vi "Pot to Degrees.vi"(11 "Pot Value":dbl) -> (3 "Degrees":dbl)   [LabVIEW 2015]
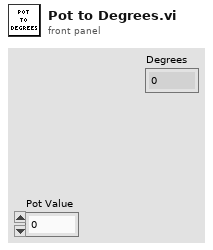
[diagram p1: front panel]
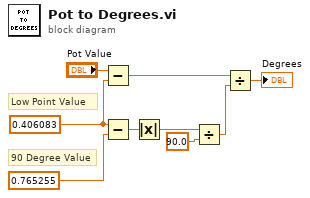
[diagram p0: block diagram]
diagram:
  w2 = 0.406083
  # "90 Degree Value"
  # "Low Point Value"
  n1 = Subtract(x="Pot Value", y=w2) -> (x-y=w7:dbl)
  n2 = Subtract(x=w2, y=0.765255) -> (x-y=w4:dbl)
  n3 = Absolute Value(x=w4) -> (abs(x)=w3:dbl)
  n4 = Divide(x=w3, y=90.0) -> (x/y=w6:dbl)
  n5 = Divide(x=w7, y=w6) -> (x/y=→"Degrees":dbl)
